vi "Sensor Mapping Example.vi"() -> ()   [LabVIEW 2016]
panel:
  in  "Data Input":bool
  in  "User-Generated":dbl[](array[slide])=[0.38383838383838387, 0.38383838383838387, 0.33333333333333337, 0.11111111111111112, 1.0] scale=0.0..1.0
  in  "stop":bool
  out "Model with Data":refnum<vi>(3d-picture)
  # "(Press LED to Toggle)"
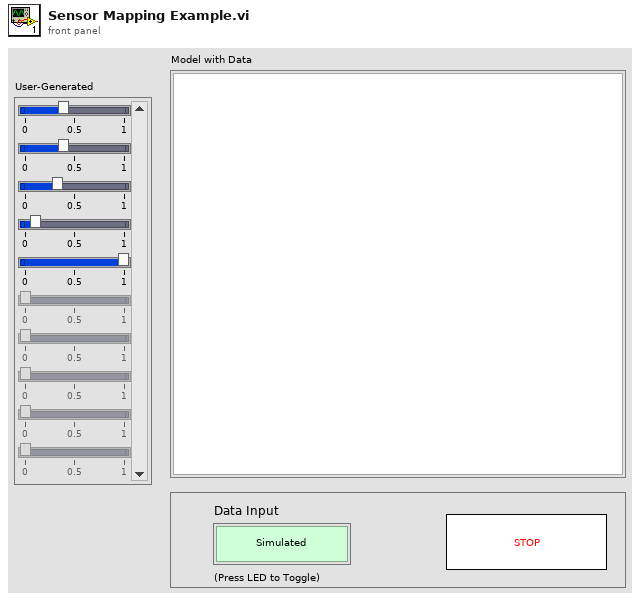
[diagram p1: front panel]
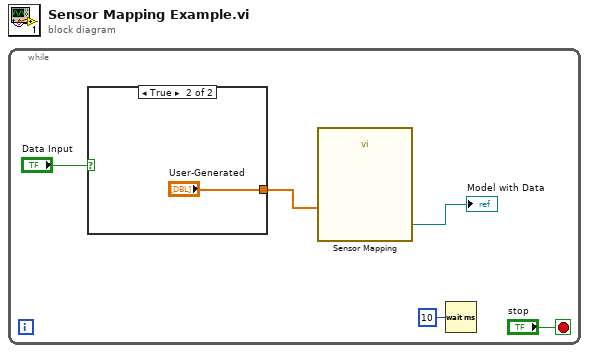
[diagram p0: block diagram]
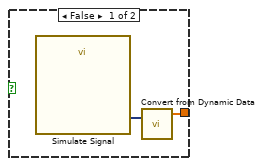
[diagram p2: hidden frame]
diagram:
  n1 = while {
    stop <- "stop" stop-if-true
    n2 = case shown="True" "Data Input" {
      tunnel: [w6 "User-Generated"] -> w2
      frame False {
        n3 = call "Simulate Signal"() -> ("Sine"=w7:dynamicdata)  [unwired: 6 in, 9 out]
        n4 = call "Convert from Dynamic Data"("Dynamic Data Type"=w7) -> ("Array"=w6:dbl[])  [unwired: 3 out]
      }
      frame True {
      }
    }
    n5 = call "Sensor Mapping"("Sensor Values"=w2) -> ("Scene Ref Out"=→"Model with Data":refnum<vi>)  [unwired: 1 in, 9 out]
    n6 = Wait (ms)(milliseconds to wait=u32 10) -> ()  [unwired: 1 out]
  }
